vi "User@ButtonBlinking__Parameter.vi"(1 "ParamterIn":string) -> (0 "ParamterOut":string)   [LabVIEW 2020]
panel:
  in  "Logic":string(combo)="ON"
  in  "UserPanelControl":string(combo)
  in  "Confirm":bool
  # "User@ButtonBlinking $UserPanelControlName,$Logic"
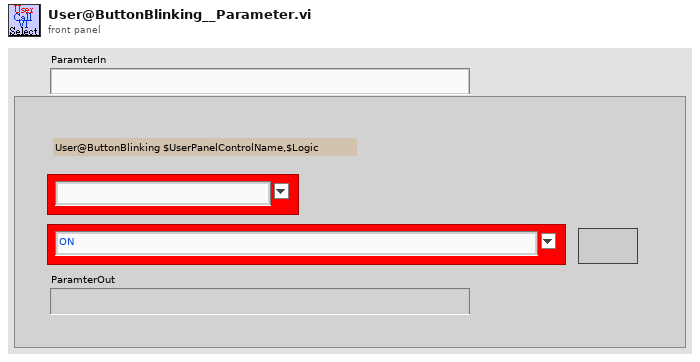
[diagram p1: front panel]
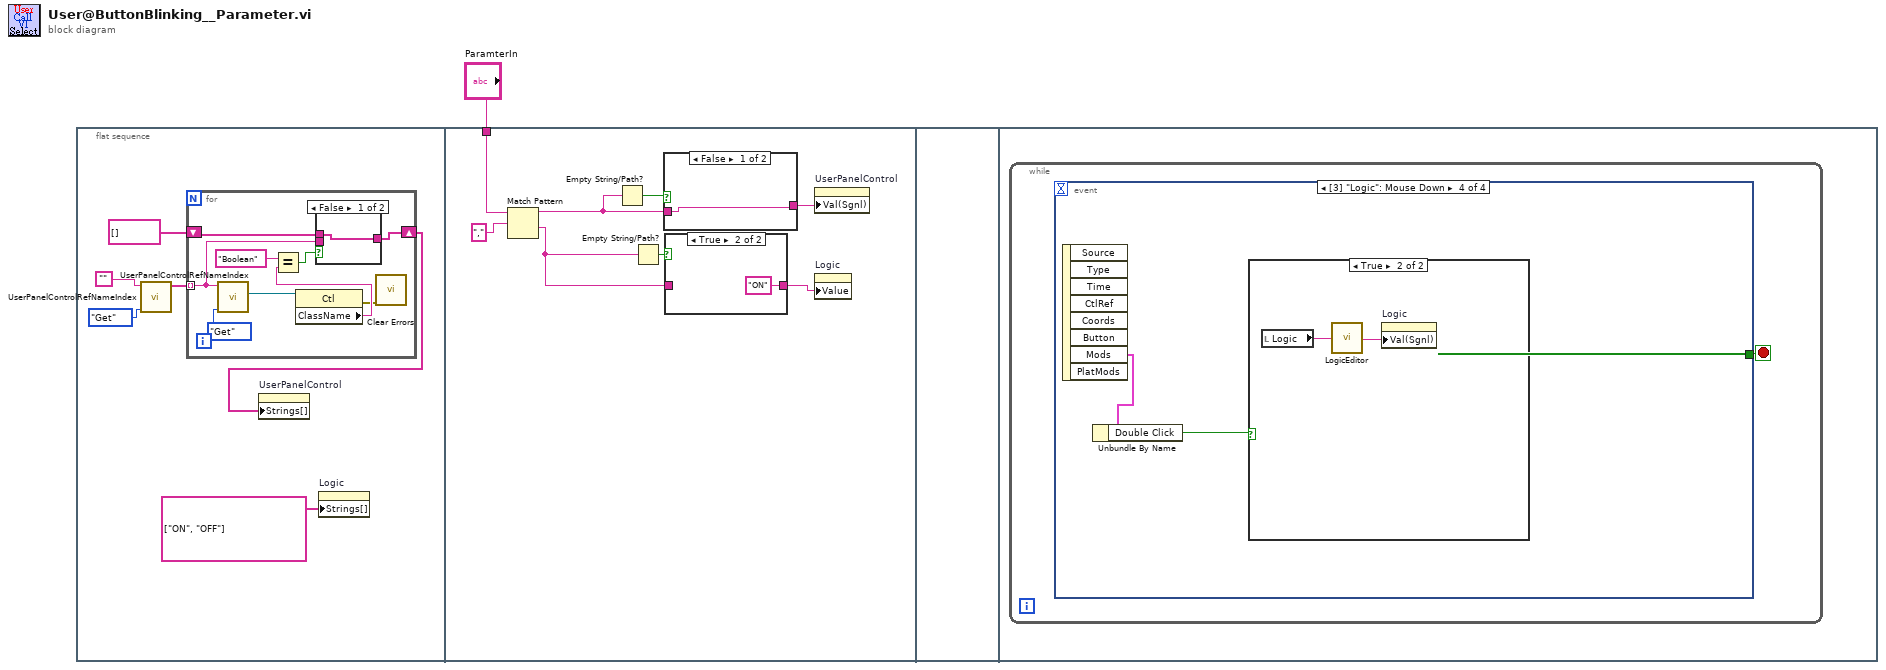
[diagram p0: block diagram]
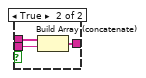
[diagram p2: hidden frame]
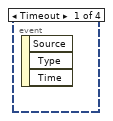
[diagram p5: hidden frame]
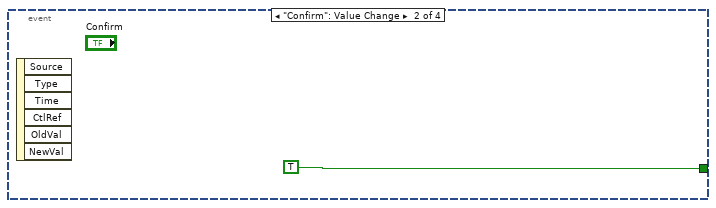
[diagram p6: hidden frame]
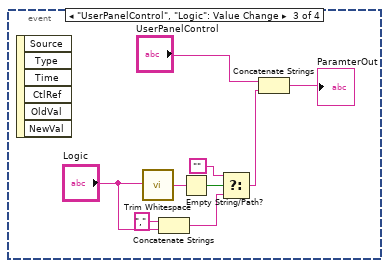
[diagram p7: hidden frame]
diagram:
  n1 = flat-sequence {
    tunnel: "ParamterIn" -> [w26]
    frame #0 {
      n2 = call "UserPanelControlRefNameIndex.vi"("OP"=enum16{"Get", "Update", "Init"}."Get", "ControlName"="") -> ("ControlNameS"=w5:string[])  [unwired: 6 in, 3 out]
      n3 = for {
        tunnel: w5 -> [w10] mode=indexing
        shift-right: [w9] -> w3
        shift-left: string[] [] ("Strings []") -> [w11]
        n4 = call "UserPanelControlRefNameIndex.vi"("OP"=enum16{"Get", "Update", "Init"}."Get", "ControlName"=w10) -> ("ControlRefOut"=w15:refnum<vi>)  [unwired: 6 in, 3 out]
        n5 = property class="Ctl"(reference=w15) -> (error out=w8:errorcluster, "ClassName"=w13:string)  [unwired: 1 in, 1 out]
        n6 = Equal?(x="Boolean" ("Class Name"), y=w13) -> (x = y?=w12:bool)
        n7 = case shown="False" w12 {
          tunnel: w11 -> [w17 w20]
          tunnel: w10 -> [_ w19]
          tunnel: [w17 w18] -> w9
          frame False {
          }
          frame True {
            n8 = Build Array (concatenate)(w20, w19) -> (w18:string[])
          }
        }
        n9 = call <vilib>:"Clear Errors.vi"("error in (no error)"=w8) -> ()  [unwired: 5 in, 2 out]
      }
      n10 = property on="UserPanelControl" class="CmbBox"("Strings[]"=w3) -> ()  [unwired: 2 in, 2 out]
      n11 = property on="Logic" class="CmbBox"("Strings[]"=string[] ["ON", "OFF"] ("Strings []")) -> ()  [unwired: 2 in, 2 out]
    }
    frame #1 {
      n12 = Match Pattern(string=w26, regular expression=",") -> (before substring=w24:string, after substring=w23:string)  [unwired: 1 in, 2 out]
      n13 = Empty String/Path?(string/path=w24) -> (empty?=w28:bool)
      n14 = Empty String/Path?(string/path=w23) -> (empty?=w27:bool)
      n15 = case shown="False" w28 {
        tunnel: w24 -> [w31 w32]
        tunnel: [w31 w32] -> w21
        frame False {
        }
        frame True {
        }
      }
      n16 = case shown="True" w27 {
        tunnel: [w29 "ON" ("ParamterIn")] -> w22
        tunnel: w23 -> [w29 _]
        frame False {
        }
        frame True {
        }
      }
      n17 = property on="UserPanelControl" class="CmbBox"("Val(Sgnl)"=w21) -> ()  [unwired: 2 in, 2 out]
      n18 = property on="Logic" class="CmbBox"("Value"=w22) -> ()  [unwired: 2 in, 2 out]
    }
    frame #2 {
    }
    frame #3 {
      n19 = while {
        stop <- w33 stop-if-true
        n20 = event shown="[3] \"Logic\": Mouse Down" {
          selector: _ -> [_ _ _ _]
          dyn-events: _ -> [_ _ _ _]
          timeout: _ -> [_ _ _ _]
          tunnel: [_ TRUE _ _] -> w33
          event Timeout {
            n21 = event-data() -> ()  [unwired: 1 in, 3 out]
          }
          event "Confirm": Value Change {
            n22 = event-data() -> ()  [unwired: 1 in, 6 out]
          }
          event "UserPanelControl", "Logic": Value Change {
            n23 = event-data() -> ()  [unwired: 1 in, 6 out]
            n24 = call <vilib>:"Trim Whitespace.vi"("string"="Logic") -> ("trimmed string"=w39:string)  [unwired: 1 in]
            n25 = Concatenate Strings("," ("string"), "Logic") -> (w38:string)
            n26 = Empty String/Path?(string/path=w39) -> (empty?=w40:bool)
            n27 = Select(t="", s=w40, f=w38) -> (s? t:f=w35:string)
            n28 = Concatenate Strings("UserPanelControl", w35) -> (→"ParamterOut":string)
          }
          event "Logic": Mouse Down {
            n29 = event-data() -> ("Mods"=w45:cluster{"Double Click":bool, "Menu Key":bool})  [unwired: 1 in, 7 out]
            n30 = Unbundle By Name(w45) -> ("Double Click"=w44:bool)
            n31 = case shown="True" w44 {
              frame False {
              }
              frame True {
                n32 = local read "Logic"() -> (w47:string)
                n33 = call "LogicEditor.vi"("Logic Express"=w47) -> ("LogicExpressOut"=w46:string)
                n34 = property on="Logic" class="CmbBox"("Val(Sgnl)"=w46) -> ()  [unwired: 2 in, 2 out]
              }
            }
          }
        }
      }
    }
  }
